vi "scale.vi"(8 "error in":errorcluster caption="entrée d'erreur", 9 "X":string[][](array[string]), 10 "Type X":T1(ring), 11 "scale":T3={"axis"=0, "with_mean"=TRUE, "with_std"=TRUE, "copy"=TRUE}) -> (0 "error out":errorcluster caption="sortie d'erreur", 3 "Data":T2)   [LabVIEW 2020]
doc: "Standardize a dataset along any axis\n\nCenter to the mean and component wise scale to unit variance.\n\n\nParameters :\n\n- X : {array-like, sparse matrix}\nThe data to center and scale.\n\n- axis : int (0 by default)\naxis used to compute the means and standard deviations along. If 0, independently standardize each feature, otherwise (if 1) standardize each sample.\n\n- with_mean : boolean, True by default\nIf True, center the data before scaling.\n\n- with_std : boolean, True by default\nIf True, scale the data to unit variance (or equivalently, unit standard deviation).\n\n- copy : boolean, optional, default True\nset to False to perform inplace row normalization and avoid a copy (if the input is already a numpy array or a scipy.sparse CSC matrix and if axis is 1)."
uses:
  scale.lvclass
panel:
  out "scale.lvclass":refnum<class "scale.lvclass">
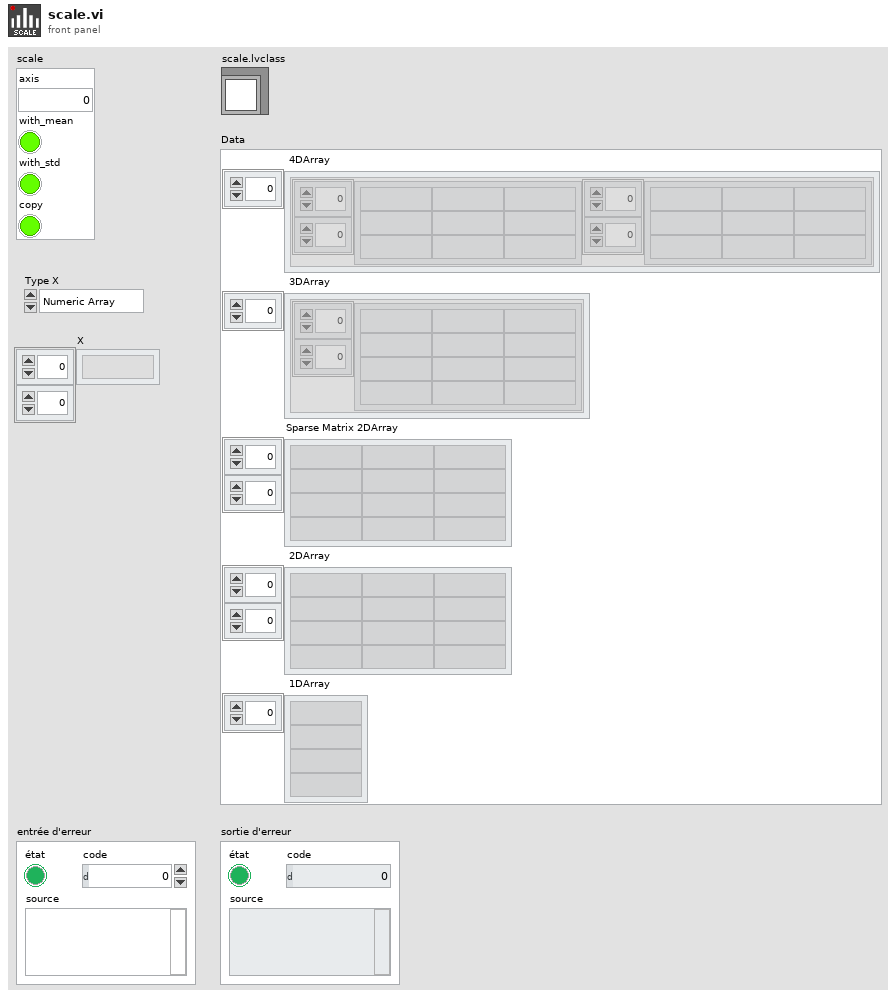
[diagram p1: front panel]
types:
  T1 = enum16{"Numeric Array", "String Array", "Sparse"}
  T2 = cluster{" 4DArray":cluster{"1":string[][], "2":string[][]}[], " 3DArray":cluster{"Tableau":string[][]}[], "Sparse Matrix 2DArray":string[][], " 2DArray":string[][], " 1DArray":string[]}
  T3 = cluster{"axis":i32, "with_mean":bool, "with_std":bool, "copy":bool}
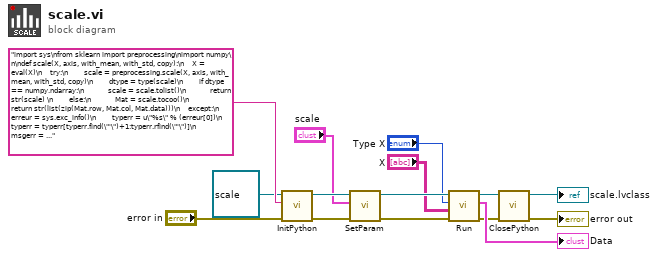
[diagram p0: block diagram]
diagram:
  n1 = call-dynamic "InitPython.vi"("error in (no error)"="error in", "Python Instruction"="import sys\nfrom sklearn import preprocessing\nimport numpy\n\ndef scale(X, axis, with_mean, with_std, copy):\n    X = eval(X)\n    try:\n        scale = preprocessing.scale(X, axis, with_mean, with_std, copy)\n        dtype = type(scale)\n        if dtype == numpy.ndarray:\n            scale = scale.tolist()\n            return str(scale) \n        else:\n            Mat = scale.tocoo()\n            return str(list(zip(Mat.row, Mat.col, Mat.data)))\n    except:\n        erreur = sys.exc_info()\n        typerr = u\"%s\" % (erreur[0])\n        typerr = typerr[typerr.find(\"'\")+1:typerr.rfind(\"'\")]\n        msgerr = u\"%s\" % (erreur[1])\n        message = str('/!\\\\ {0} : {1}'. format(typerr,msgerr))\n        return message", "Scikit-learn en entrée"=refnum<class "scale.lvclass"> refnum ("scale.lvclass")) -> ("error out"=w8:errorcluster, "Scikit-learn en sortie"=w10:refnum<class "scale.lvclass">)  [unwired: 7 in]
  n2 = call-dynamic "SetParam.vi"("error in (no error)"=w8, "scale"="scale", "scale.lvclass"=w10) -> ("error out"=w5:errorcluster, "scale.lvclass"=w7:refnum<class "scale.lvclass">)  [unwired: 7 in]
  n3 = call-dynamic "Run.vi"("error in (no error)"=w5, "X"="X", "Type X"="Type X", "scale.lvclass"=w7) -> ("error out"=w2:errorcluster, "Data"=→"Data":T2, "scale.lvclass"=w4:refnum<class "scale.lvclass">)  [unwired: 5 in]
  n4 = call-dynamic "ClosePython.vi"("error in (no error)"=w2, "Scikit-learn en entrée"=w4) -> ("error out"=→"error out":errorcluster, "Scikit-learn en sortie"=→"scale.lvclass":refnum<class "scale.lvclass">)  [unwired: 8 in]
